vi "ParseError.vi"(8 "error in (no error)":errorcluster, 11 "GRMActor in":refnum<class "GeneralRMActor.lvclass">) -> (0 "error out":errorcluster, 3 "GRMActor out":refnum<class "GeneralRMActor.lvclass">)   [LabVIEW 2020, in "GeneralRMActor.lvlib" / "GeneralRMActor.lvclass"]
uses:
  GeneralRMActor.lvclass
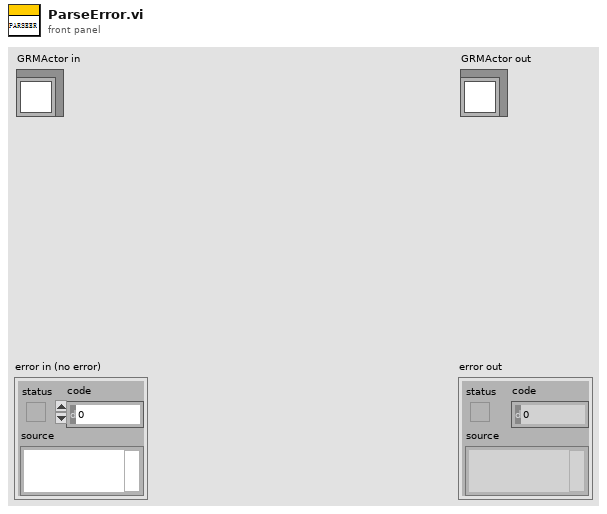
[diagram p1: front panel]
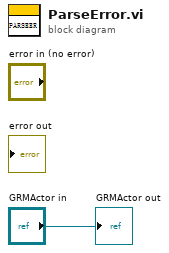
[diagram p0: block diagram]
diagram:
  "GRMActor out" <- "GRMActor in"
